vi "Get Color.vi"(11 "Blue Plugin in":refnum<class "Blue Plugin.lvclass">) -> (3 "Color Box":u32(colorbox))   [LabVIEW 2014, in "Blue Plugin.lvclass"]
uses:
  Blue Plugin.lvclass
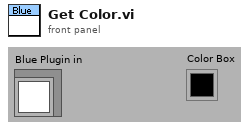
[diagram p1: front panel]
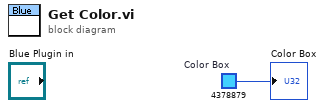
[diagram p0: block diagram]
diagram:
  w1 = u32 4378879  # Color Box
  "Color Box" <- w1
